vi "SetFloatValue.vi"(8 "error in (no error)":errorcluster caption="错误输入（无错误）", 9 "fValue":sgl, 10 "strValue":string, 11 "handle":u64) -> (0 "error out":errorcluster caption="错误输出", 2 "function return":i32, 3 "handle out":u64)   [LabVIEW 2015, in "MvCameraControl.lvlib"]
doc: "MV_LV_API int __stdcall SetFloatValue( void* handle, const char* strValue, float fValue);"
uses:
  MvCameraControl.lvlib
  MvCameraControl.dll
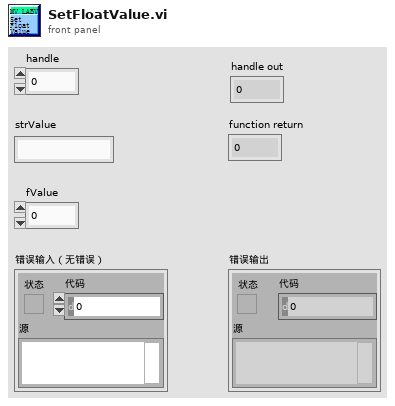
[diagram p1: front panel]
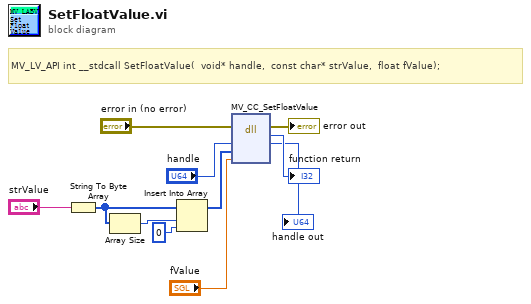
[diagram p0: block diagram]
diagram:
  # "MV_LV_API int __stdcall SetFloatValue(  void* handle,  const char* strValue,  float fValue);"
  n1 = String To Byte Array(string="strValue") -> (unsigned byte array=w6:u8[])
  n2 = Array Size(array=w6) -> (size(s)=w5:i32)
  n3 = Insert Into Array(array=w6, index=w5, new element=u8 0 ("新元素/子数组")) -> (w2:u8[])
  n4 = dll-call lib="MvCameraControl.dll" fn="MV_CC_SetFloatValue"(error in="error in (no error)", "handle"="handle", "strKey"=w2, "fValue"="fValue") -> (error out=→"error out":errorcluster, "返回类型"=→"function return":i32, "handle"=→"handle out":u64)  [unwired: 4 in, 1 out]
